vi "SavePic.vi"() -> ()   [LabVIEW 2012]
panel:
  in  "Save":bool
  in  "vi path":path
  in  "Select Path (dialog if empty) 2":path
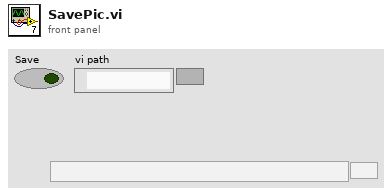
[diagram p1: front panel]
types:
  T1 = typedef "imagedata.ctl" = cluster{"image type":i32, "image depth":i32, "image":u8[], "mask":u8[], "colors":u32[], "Rectangle":cluster{"left":i16, "top":i16, "right":i16, "bottom":i16}}
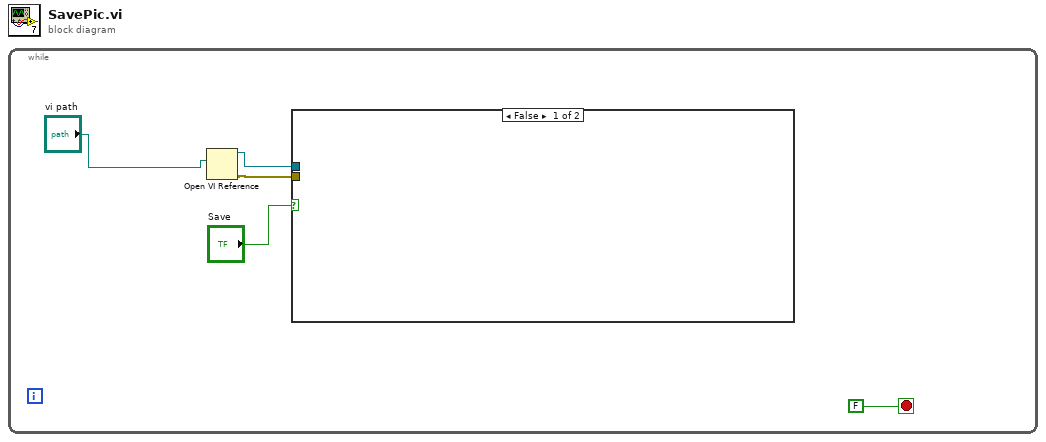
[diagram p0: block diagram]
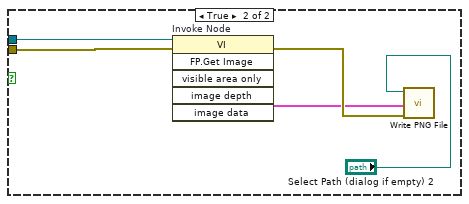
[diagram p2: hidden frame]
diagram:
  n1 = while {
    stop <- FALSE ("stop") stop-if-true
    n2 = Open VI Reference(vi path="vi path") -> (vi reference=w2:refnum<vi>, error out=w1:errorcluster)  [unwired: 5 in]
    n3 = case shown="False" "Save" {
      tunnel: w2 -> [_ w7]
      tunnel: w1 -> [_ w6]
      frame False {
      }
      frame True {
        n4 = invoke on="Invoke Node" class="VI" method="FP.Get Image"(reference=w7, error in=w6) -> (error out=w10:errorcluster, "image data"=w8:T1)  [unwired: 4 in, 4 out]
        n5 = call <vilib>:"Write PNG File.vi"("error in (no error)"=w10, "image data"=w8, "path to PNG file"="Select Path (dialog if empty) 2") -> ()  [unwired: 9 out]
      }
    }
  }
